vi "Actualizar_Interfaz.vi"(8 "error in (no error)":errorcluster, 10 "Enum":T1, 11 "Controls":refnum<vi>[](array[refnum])) -> (0 "error out":errorcluster, 3 "Controls 2":refnum<vi>[](array[refnum]))   [LabVIEW 2019, in "SHARED VI'S.lvlib"]
uses:
  SHARED VI'S.lvlib
  SHARED TYPES/Acciones_UI.ctl
  SHARED TYPES/SHARED TYPES.lvlib
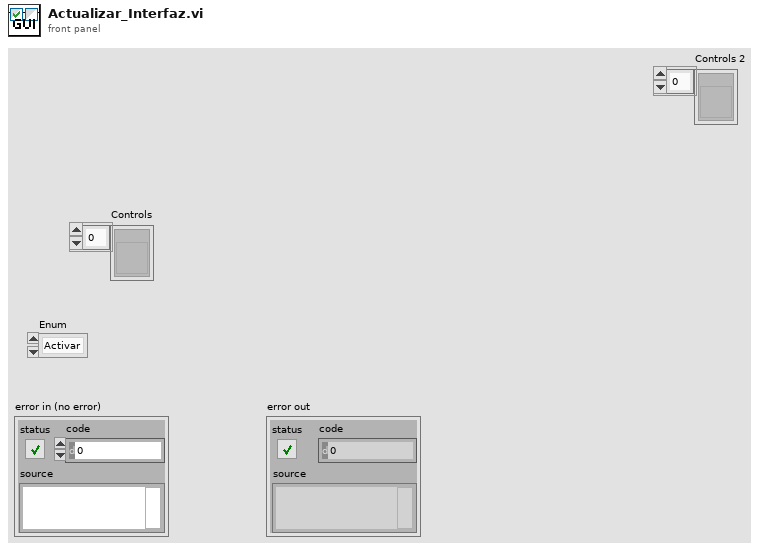
[diagram p1: front panel]
types:
  T1 = typedef "SHARED TYPES.lvlib/Acciones_UI.ctl" = enum16{"Activar", "Desactivar", "Reiniciar default"}
  T2 = enum8{"Enabled", "Disabled", "Disabled and Grayed Out"}
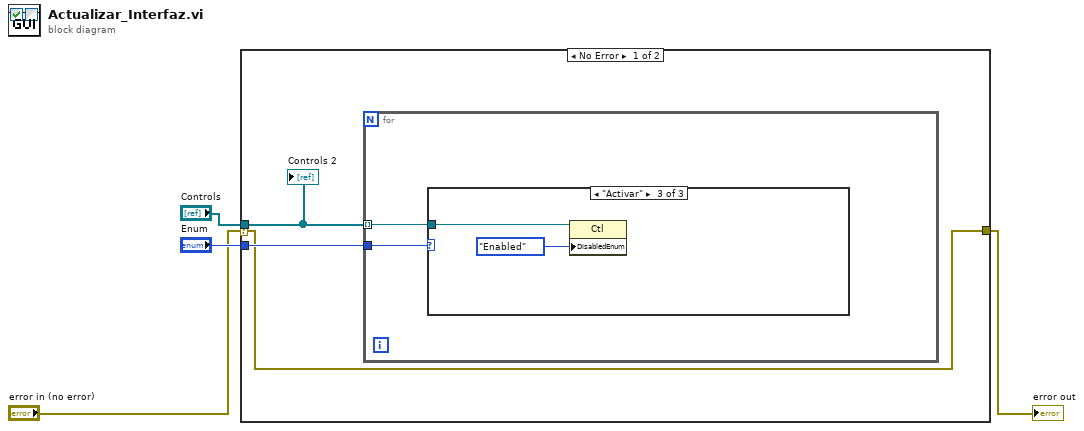
[diagram p0: block diagram]
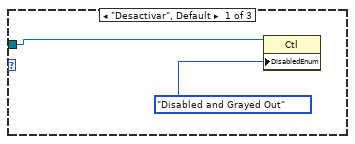
[diagram p2: hidden frame]
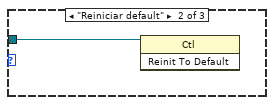
[diagram p3: hidden frame]
diagram:
  n1 = case shown="No Error" "error in (no error)" {
    selector: "error in (no error)" -> [w5 w15]
    tunnel: "Enum" -> [w7 _]
    tunnel: "Controls" -> [w6 _]
    tunnel: [w5 w15] -> w1
    frame No Error {
      n2 = for {
        tunnel: w7 -> [w9]
        tunnel: w6 -> [w8] mode=indexing
        n3 = case shown="\"Activar\"" w9 {
          tunnel: w8 -> [w10 w12 w13]
          frame "Desactivar", Default {
            n4 = property class="Ctl"(reference=w10, "DisabledEnum"=T2."Disabled and Grayed Out" ("Disabled")) -> ()  [unwired: 1 in, 2 out]
          }
          frame "Reiniciar default" {
            n5 = invoke class="Ctl" method="Reinit To Default"(reference=w12) -> ()  [unwired: 2 in, 3 out]
          }
          frame "Activar" {
            n6 = property class="Ctl"(reference=w13, "DisabledEnum"=T2."Enabled" ("Disabled")) -> ()  [unwired: 1 in, 2 out]
          }
        }
      }
      "Controls 2" <- w6
    }
    frame Error {
    }
  }
  "error out" <- w1
